vi "ESP301_Read_Position.vi"(10 "axisNumber":i32=1, 11 "COM_PORT":string="COM12") -> (0 "errstring":string, 1 "MD":bool, 2 "Motor_status":bool, 3 "Position":dbl, 8 "Error":bool)   [LabVIEW 2019]
uses:
  Newport.ESP301.CommandInterface
panel:
  out "MD":i32
  out "errstring 3":string
  out "errstring 2":string
  out "MO_Get":i32
  out "TP":i32
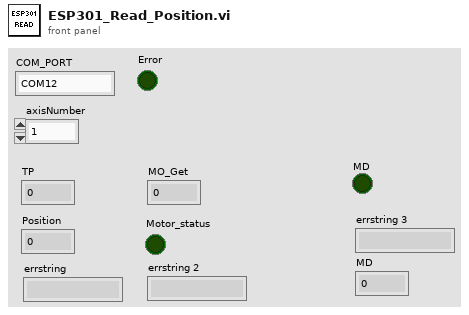
[diagram p1: front panel]
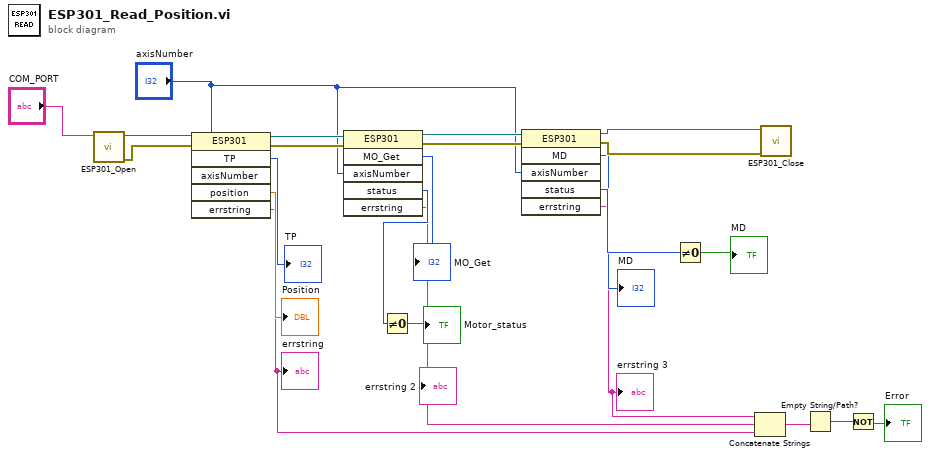
[diagram p0: block diagram]
diagram:
  n1 = call "ESP301_Open.vi"("strDeviceKey"="COM_PORT") -> ("sortie d'erreur"=w21:errorcluster, "référence en sortie"=w22:refnum<k24>)  [unwired: 9 in]
  n2 = invoke on="Nœud de méthode" class="ESP301" method="TP"(reference=w22, error in=w21, "axisNumber"="axisNumber") -> (reference out=w24:refnum<k24>, error out=w23:errorcluster, "TP"=→"TP":i32, "position"=→"Position":dbl, "errstring"=w4:string)  [unwired: 3 in, 1 out]
  "errstring" <- w4
  n3 = invoke on="Nœud de méthode" class="ESP301" method="MO_Get"(reference=w24, error in=w23, "axisNumber"="axisNumber") -> (reference out=w14:refnum<k24>, error out=w13:errorcluster, "MO_Get"=→"MO_Get":i32, "status"=w17:i32, "errstring"=w5:string)  [unwired: 3 in, 1 out]
  "errstring 2" <- w5
  n4 = Not Equal To 0?(x=w17) -> (x != 0?=→"Motor_status":bool)
  n5 = invoke on="Nœud de méthode" class="ESP301" method="MD"(reference=w14, error in=w13, "axisNumber"="axisNumber") -> (reference out=w12:refnum<k24>, error out=w11:errorcluster, "MD"=→"MD":i32, "status"=w9:i32, "errstring"=w6:string)  [unwired: 3 in, 1 out]
  "errstring 3" <- w6
  n6 = Not Equal To 0?(x=w9) -> (x != 0?=→"MD":bool)
  n7 = Concatenate Strings(w6, w5, w4) -> (w3:string)
  n8 = call "ESP301_Close.vi"("entrée d'erreur (pas d'erreur)"=w11, "référence"=w12) -> ()  [unwired: 9 in, 1 out]
  n9 = Empty String/Path?(string/path=w3) -> (empty?=w1:bool)
  n10 = Not(x=w1) -> (.not. x?=→"Error":bool)
